vi "Threshold Detection (SubVI).vi"(9 "Array 2":dbl[](array[numeric]), 10 "index":i32, 11 "Array":dbl[](array[numeric])) -> (3 "Output":dbl)   [LabVIEW 2026]
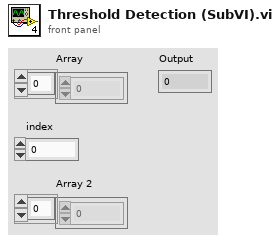
[diagram p1: front panel]
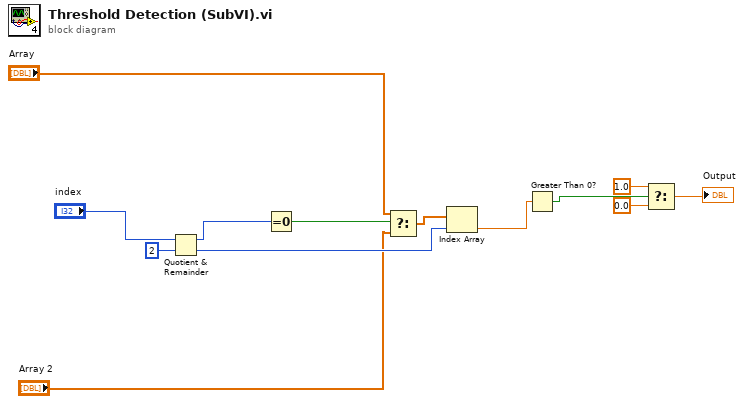
[diagram p0: block diagram]
diagram:
  n1 = Quotient & Remainder(x="index", y=2) -> (x-y*floor(x/y)=w3:i32, floor(x/y)=w8:i32)
  n2 = Equal To 0?(x=w3) -> (x = 0?=w5:bool)
  n3 = Select(t="Array", s=w5, f="Array 2") -> (s? t:f=w7:dbl[])
  n4 = Index Array(array=w7, index=w8) -> (element=w9:dbl)
  n5 = Greater Than 0?(x=w9) -> (x > 0?=w10:bool)
  n6 = Select(t=1.0, s=w10, f=0.0) -> (s? t:f=→"Output":dbl)
